vi "题目3.vi"() -> ()   [LabVIEW 2017]
panel:
  out "字符串":string
  in  "停止":bool
  in  "布尔":bool
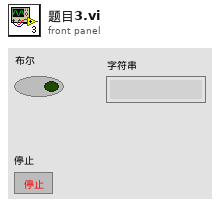
[diagram p1: front panel]
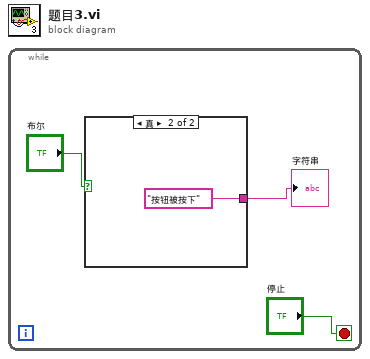
[diagram p0: block diagram]
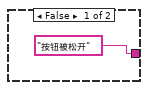
[diagram p2: hidden frame]
diagram:
  n1 = while {
    stop <- "停止" stop-if-true
    n2 = case shown="真" "布尔" {
      tunnel: ["按钮被松开" "按钮被按下"] -> w2
      frame False {
      }
      frame True {
      }
    }
    "字符串" <- w2
  }
